vi "Unregister PVs.vi"(8 "error in (no error)":errorcluster, 10 "Unegister Info":T1, 11 "CS++PVMonitor in":refnum<class "CS++PVMonitor.lvclass">) -> (0 "error out":errorcluster, 3 "CS++PVMonitor out":refnum<class "CS++PVMonitor.lvclass">)   [LabVIEW 2012, in "CS++PVMonitor.lvlib" / "CS++PVMonitor.lvclass"]
doc: "Unregister process variables."
uses:
  CS++PVMonitor.lvclass
  <vilib>/ActorFramework/Message Enqueuer/Message Enqueuer.lvclass
  CS++PVMonitor.lvclass/CS++PVMonitor.ctl
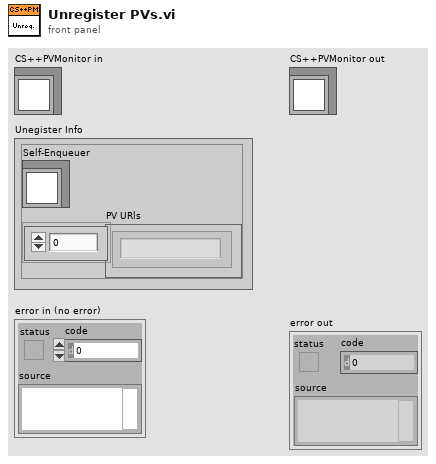
[diagram p1: front panel]
types:
  T1 = cluster{"Self-Enqueuer":refnum<class "Message Enqueuer.lvclass">, "PV URls":string[]}
  T2 = cluster{"PV URL":string, "Observers":cluster{"Enqueuer":refnum<class "Message Enqueuer.lvclass">, "CS++PVUpdate Msg":refnum<class "CS++PVUpdate Msg.lvclass">}[]}[]
  T3 = cluster{"PV URL":string, "Observers":cluster{"Enqueuer":refnum<class "Message Enqueuer.lvclass">, "CS++PVUpdate Msg":refnum<class "CS++PVUpdate Msg.lvclass">}[]}
  T4 = cluster{"Enqueuer":refnum<class "Message Enqueuer.lvclass">, "CS++PVUpdate Msg":refnum<class "CS++PVUpdate Msg.lvclass">}[]
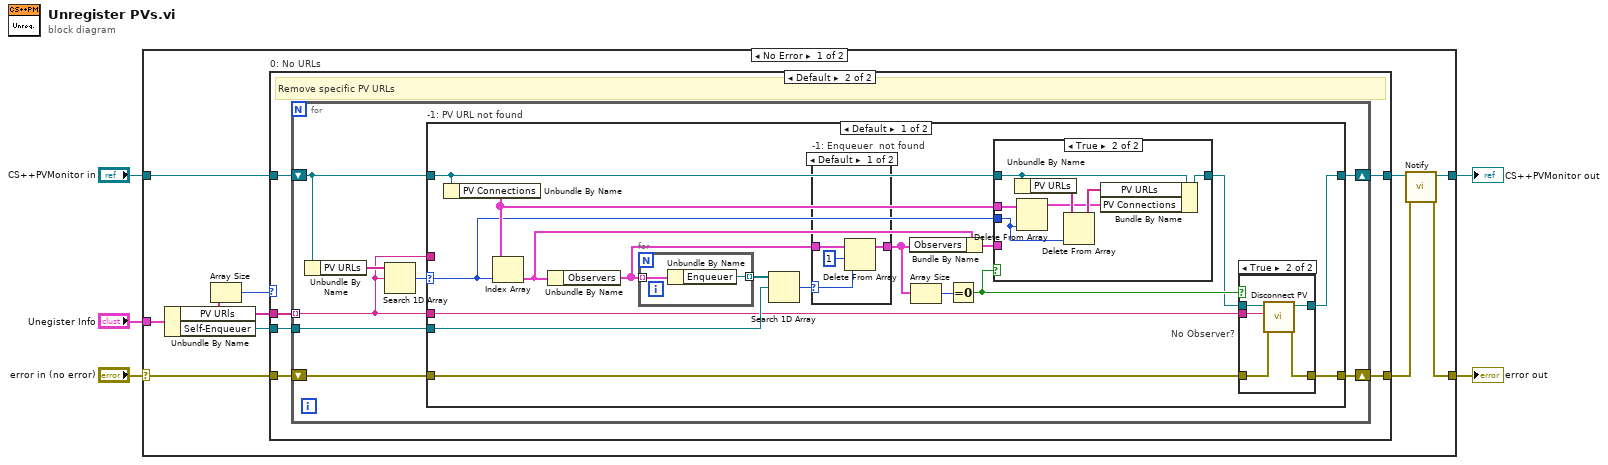
[diagram p0: block diagram]
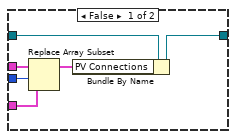
[diagram p3: hidden frame]
diagram:
  n1 = case shown="No Error" "error in (no error)" {
    selector: "error in (no error)" -> [w14 w79]
    tunnel: [w7 w79] -> w1
    tunnel: [w8 w78] -> w2
    tunnel: "CS++PVMonitor in" -> [w13 w78]
    tunnel: "Unegister Info" -> [w15 _]
    frame No Error {
      n2 = Unbundle By Name(w15) -> ("PV URls"=w11:string[], "Self-Enqueuer"=w12:refnum<class "Message Enqueuer.lvclass">)
      n3 = Array Size(array=w11) -> (size(s)=w10:i32)
      n4 = case "0: No URLs" shown="Default" w10 {
        tunnel: w11 -> [_ w23]
        tunnel: w14 -> [w16 w22]
        tunnel: [w16 w21] -> w6
        tunnel: w13 -> [w17 w20]
        tunnel: [w17 w19] -> w9
        tunnel: w12 -> [_ w18]
        frame 0 {
          # "Remove observer from all PV URLs; to be implemented!"
        }
        frame Default {
          # "Remove specific PV URLs"
          n5 = for {
            tunnel: w23 -> [w24] mode=indexing
            shift-right: [w26] -> w21
            shift-left: w22 -> [w25]
            shift-right: [w27] -> w19
            shift-left: w20 -> [w29]
            tunnel: w18 -> [w28]
            n6 = Unbundle By Name(w29) -> ("PV URLs"=w31:string[])
            n7 = Search 1D Array(1D array=w31, element=w24) -> (index of element=w30:i32)  [unwired: 1 in]
            n8 = case "-1: PV URL not found" shown="Default" w30 {
              selector: w30 -> [w45 _]
              tunnel: w29 -> [w33 w77]
              tunnel: w28 -> [w43 _]
              tunnel: w24 -> [w36 _]
              tunnel: [w39 w77] -> w27
              tunnel: [w37 w76] -> w26
              tunnel: w25 -> [w38 w76]
              tunnel: w24 -> [_ _]
              frame Default {
                n9 = Unbundle By Name(w33) -> ("PV Connections"=w46:T2)
                n10 = Index Array(array=w46, index=w45) -> (element=w44:T3)
                n11 = Unbundle By Name(w44) -> ("Observers"=w47:T4)
                n12 = for {
                  tunnel: w47 -> [w75] mode=indexing
                  tunnel: [w74] -> w48 mode=indexing
                  n13 = Unbundle By Name(w75) -> ("Enqueuer"=w74:refnum<class "Message Enqueuer.lvclass">)
                }
                n14 = Search 1D Array(1D array=w48, element=w43) -> (index of element=w41:i32)  [unwired: 1 in]
                n15 = case "-1: Enqueuer  not found" shown="Default" w41 {
                  selector: w41 -> [w70 _]
                  tunnel: w47 -> [w72 w73]
                  tunnel: [w71 w73] -> w40
                  frame Default {
                    n16 = Delete From Array(array=w72, length=1, index=w70) -> (array with subset deleted=w71:T4)  [unwired: 1 out]
                  }
                  frame -1 {
                  }
                }
                n17 = Bundle By Name(cluster=w44, "Observers"=w40) -> (w42:T3)
                n18 = Array Size(array=w40) -> (size(s)=w35:i32)
                n19 = Equal To 0?(x=w35) -> (x = 0?=w34:bool)
                n20 = case shown="True" w34 {
                  tunnel: w46 -> [w54 w61]
                  tunnel: w45 -> [w53 w59]
                  tunnel: w42 -> [w52 _]
                  tunnel: w33 -> [w51 w58]
                  tunnel: [w50 w56] -> w32
                  frame False {
                    n21 = Replace Array Subset(array=w54, new element=w52, index=w53) -> (w49:T2)
                    n22 = Bundle By Name(cluster=w51, "PV Connections"=w49) -> (w50:refnum<class "CS++PVMonitor.lvclass">)
                  }
                  frame True {
                    n23 = Unbundle By Name(w58) -> ("PV URLs"=w60:string[])
                    n24 = Delete From Array(array=w61, index=w59) -> (array with subset deleted=w55:T2)  [unwired: 1 in, 1 out]
                    n25 = Delete From Array(array=w60, index=w59) -> (array with subset deleted=w57:string[])  [unwired: 1 in, 1 out]
                    n26 = Bundle By Name(cluster=w58, "PV URLs"=w57, "PV Connections"=w55) -> (w56:refnum<class "CS++PVMonitor.lvclass">)
                  }
                }
                n27 = case "No Observer?" shown="True" w34 {
                  tunnel: w32 -> [w63 w68]
                  tunnel: [w63 w67] -> w39
                  tunnel: w38 -> [w62 w66]
                  tunnel: [w62 w65] -> w37
                  tunnel: w36 -> [_ w64]
                  frame False {
                  }
                  frame True {
                    n28 = call-dynamic "Disconnect PV.vi"("error in (no error)"=w66, "PV URL"=w64, "CS++PVMonitor in"=w68) -> ("error out"=w65:errorcluster, "CS++PVMonitor out"=w67:refnum<class "CS++PVMonitor.lvclass">)  [unwired: 7 in]
                  }
                }
              }
              frame -1 {
              }
            }
          }
        }
      }
      n29 = call-dynamic "Notify.vi"("error in (no error)"=w6, "CS++PVMonitor in"=w9) -> ("error out"=w7:errorcluster, "CS++PVMonitor out"=w8:refnum<class "CS++PVMonitor.lvclass">)  [unwired: 8 in]
    }
    frame Error {
    }
  }
  "error out" <- w1
  "CS++PVMonitor out" <- w2
